vi "Pause_fcn (SubVI).vi"(10 "Eta":dbl[](array[numeric]), 11 "Eta_des":dbl[](array[numeric])) -> (2 "Go":bool, 3 "Pause":bool)   [LabVIEW 2014, in "Guidance Library.lvlib" / "Constant Jerk Guidance.lvclass"]
uses:
  Constant Jerk Guidance.lvclass
panel:
  in  "tol":dbl=1.5
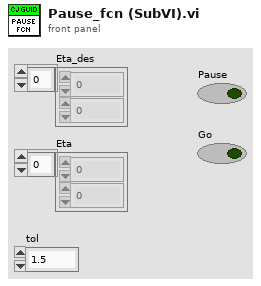
[diagram p1: front panel]
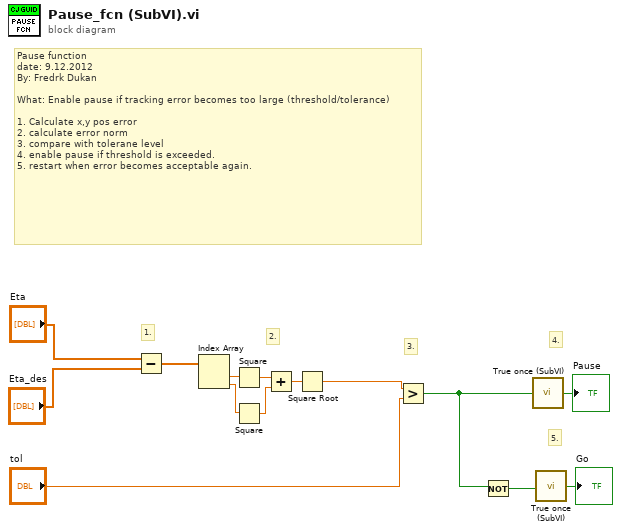
[diagram p0: block diagram]
diagram:
  # "5."
  # "Pause function                                                                                                \ndate: 9.12.2012\nBy: Fredrk Dukan\n\nWhat: Enable pause if tracking error becomes too large (threshold/tolerance)\n\n1. Calculate x,y pos error\n2. calculate error norm\n3. compare with tolerane level\n4. enable pause if threshold is exceeded.\n5. restart when error becomes acceptable again."
  # "4."
  # "3."
  # "2."
  # "1."
  n1 = Subtract(x="Eta", y="Eta_des") -> (x-y=w12:dbl[])
  n2 = Index Array(array=w12) -> (element #1=w11:dbl, element #2=w10:dbl)  [unwired: 2 in]
  n3 = Square(x=w11) -> (x^2=w9:dbl)
  n4 = Square(x=w10) -> (x^2=w8:dbl)
  n5 = Add(x=w9, y=w8) -> (x+y=w7:dbl)
  n6 = Square Root(x=w7) -> (sqrt(x)=w6:dbl)
  n7 = Greater?(x=w6, y="tol") -> (0:w4:bool)
  n8 = Not(x=w4) -> (.not. x?=w3:bool)
  n9 = call "True once (SubVI).vi"("Automatic"=w4) -> ("Boolean"=→"Pause":bool)
  n10 = call "True once (SubVI).vi"("Automatic"=w3) -> ("Boolean"=→"Go":bool)
